vi "Write Elements of HTML-PDF-&allTempNames.vi"(8 "error in (no error)":errorcluster, 10 "Array":string[](array[string]), 11 "Folder_Mgmt":refnum<class "Folder_Mgmt.lvclass">) -> (0 "error out":errorcluster, 3 "Folder_Mgmt 2":refnum<class "Folder_Mgmt.lvclass">)   [LabVIEW 2016, in "Folder_Mgmt.lvclass"]
uses:
  Folder_Mgmt.lvclass
  Folder_Mgmt.lvclass/Folder_Mgmt.ctl
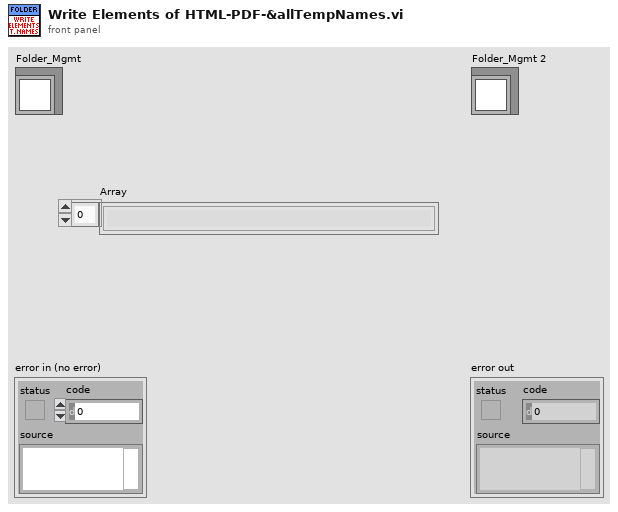
[diagram p1: front panel]
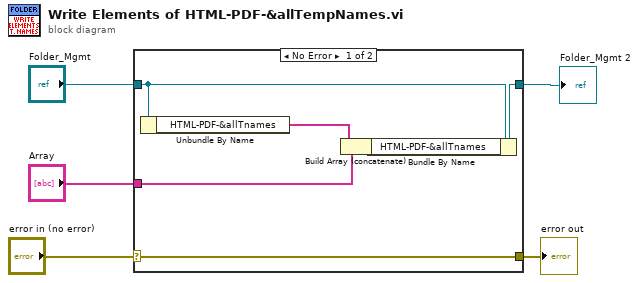
[diagram p0: block diagram]
diagram:
  n1 = case shown="No Error" "error in (no error)" {
    selector: "error in (no error)" -> [w11 w12]
    tunnel: [w11 w12] -> w4
    tunnel: [w10 w13] -> w2
    tunnel: "Folder_Mgmt" -> [w9 w13]
    tunnel: "Array" -> [w8 _]
    frame No Error {
      n2 = Unbundle By Name(w9) -> ("HTML-PDF-&allTnames"=w6:string[])
      n3 = Build Array (concatenate)(w6, w8) -> (w7:string[])
      n4 = Bundle By Name(cluster=w9, "HTML-PDF-&allTnames"=w7) -> (w10:refnum<class "Folder_Mgmt.lvclass">)
    }
    frame Error {
    }
  }
  "error out" <- w4
  "Folder_Mgmt 2" <- w2
